vi "Format Header Columns.vi"(8 "error in (no error)":errorcluster, 9 "Sort Order":i32, 10 "Sort Column":i32, 11 "Controls Table Ref":refnum<vi>) -> (0 "error out":errorcluster)   [LabVIEW 2020, in "VI Properties Editor.lvlib"]
doc: "Formats the header columns of the Controls table."
uses:
  VI Properties Editor.lvlib
  <vilib>/Utility/miscctls.llb/LVRowAndColumnTypeDef.ctl
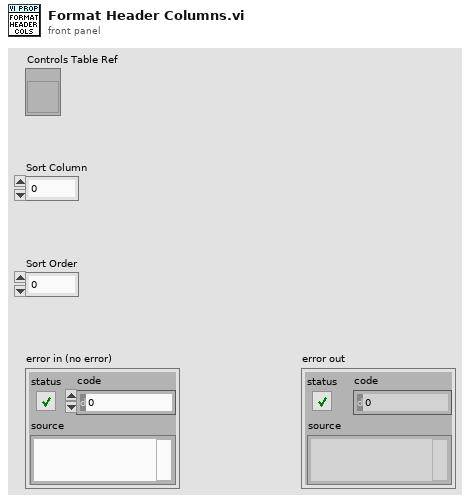
[diagram p1: front panel]
types:
  T1 = typedef "LVRowAndColumnTypeDef.ctl" = cluster{"Row":i32, "Column":i32}
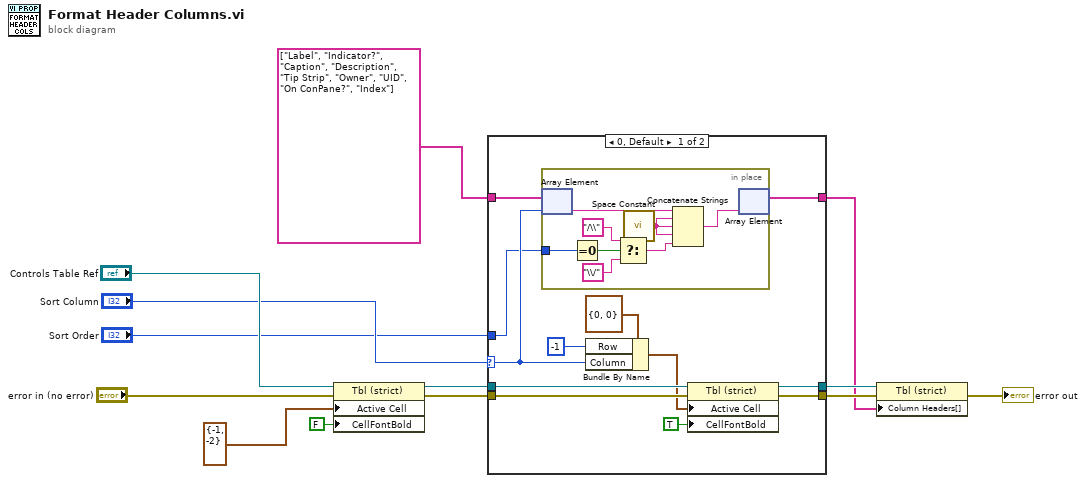
[diagram p0: block diagram]
diagram:
  n1 = property class="Tbl (strict)"(reference="Controls Table Ref", error in="error in (no error)", "Active Cell"=T1 {"Row"=-1, "Column"=-2} ("Active Cell:Active Cell"), "CellFontBold"=FALSE ("Active Cell:Cell Font:Bold")) -> (reference out=w9:refnum<vi>, error out=w8:errorcluster)
  n2 = case shown="0, Default" "Sort Column" {
    selector: "Sort Column" -> [w16 _]
    tunnel: w9 -> [w25 w35]
    tunnel: w8 -> [w24 w36]
    tunnel: [w23 w36] -> w6
    tunnel: [w18 w35] -> w5
    tunnel: string[] ["Label", "Indicator?", "Caption", "Description", "Tip Strip", "Owner", "UID", "On ConPane?", "Index"] -> [w17 w34]
    tunnel: "Sort Order" -> [w15 _]
    tunnel: [w14 w34] -> w2
    frame 0, Default {
      n3 = in-place {
        in-place-border: w15 -> [w33]
        n4 = in-place-array #1(w17, w16) -> (w32:string)
        n5 = Equal To 0?(x=w33) -> (x = 0?=w31:bool)
        n6 = Select(t="/\\", s=w31, f="\\/") -> (s? t:f=w28:string)
        n7 = call <vilib>:"Space Constant.vi"() -> ("String"=w26:string)
        n8 = Concatenate Strings(w32, w26, w26, w26, w28) -> (w27:string)
        n9 = in-place-array #1(w27) -> (w14:string[])  [unwired: 1 out]
      }
      n10 = Bundle By Name(cluster=T1 {"Row"=0, "Column"=0} ("Active Cell:Active Cell"), "Row"=-1, "Column"=w16) -> (w19:T1)
      n11 = property class="Tbl (strict)"(reference=w25, error in=w24, "Active Cell"=w19, "CellFontBold"=TRUE ("Active Cell:Cell Font:Bold")) -> (reference out=w18:refnum<vi>, error out=w23:errorcluster)
    }
    frame -1 {
    }
  }
  n12 = property class="Tbl (strict)"(reference=w5, error in=w6, "Column Headers[]"=w2) -> (error out=→"error out":errorcluster)  [unwired: 1 out]
